vi "niSYS - SA - MEAS - UTIL - 1 Ohm Voltage to Vrms (CSGL array).vi"(7 "Complex Array, V":cdb[](array[numeric]) format="%.1f") -> (8 "Real Array, dBm":dbl[](array[numeric]) format="%.3f")   [LabVIEW 2019]
doc: "(c) Copyright 2006, National Instruments, Inc. This VI may not be duplicated, sold, or distributed without written consent from National Instruments."
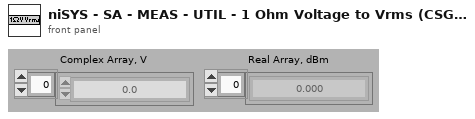
[diagram p1: front panel]
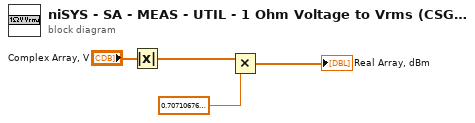
[diagram p0: block diagram]
diagram:
  n1 = Absolute Value(x="Complex Array, V") -> (abs(x)=w3:dbl[])
  n2 = Multiply(x=w3, y=0.7071067690849304 ("1/x")) -> (x*y=→"Real Array, dBm":dbl[])
